vi "Add card dialog.vi"(8 "error in (no error)":errorcluster, 9 "Card Position":T1={"Rack #"=0, "Slot #"=1} {"Slot #" max=15}, 10 "Card Type in":string, 11 "Node Ptr":u64 format="%.0x") -> (0 "error out":errorcluster, 1 "Card Position out":T1={"Rack #"=0, "Slot #"=1} {"Slot #" max=15}, 2 "Name out":string, 3 "Node Ptr out":u64 format="%.0x", 4 "Cancelled?":bool)   [LabVIEW 2014, in "SLSC configuration System Explorer.lvlib"]
uses:
  SLSC configuration System Explorer.lvlib
  Type Defs/Card Position.ctl
  Shared/SPI Utility/Slot #.ctl
  Type Defs/Valid.ctl
  Shared/Constants.vi
  <vilib>/NI Veristand/Custom Device API/Custom Device API.lvlib
  Shared/SLSC configuration Shared.lvlib
panel:
  out "Valid?":T3
  in  "Name":string
  in  "Cancel":bool
  in  "Add":bool
  out "Card Type":string
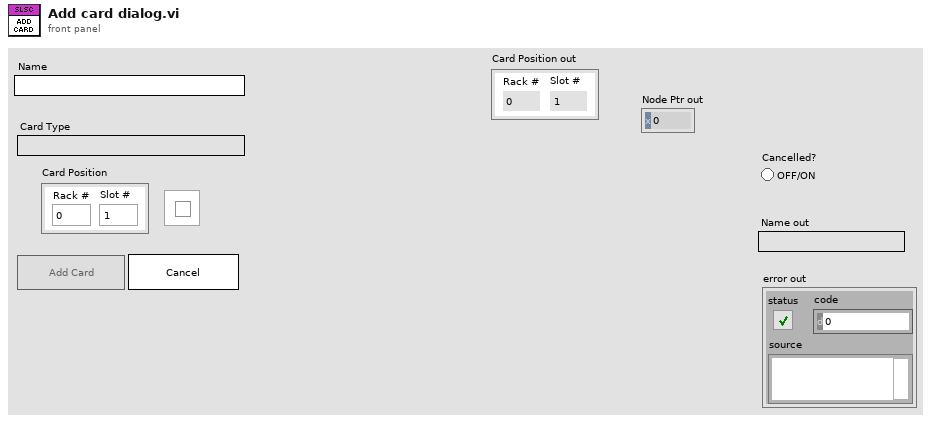
[diagram p1: front panel]
types:
  T1 = typedef "SLSC configuration Shared.lvlib/Card Position.ctl" = cluster{"Rack #":u8, "Slot #":T2}
  T2 = typedef "SLSC configuration Shared.lvlib/Slot #.ctl" = u8
  T3 = typedef "SLSC configuration System Explorer.lvlib/Valid.ctl" = bool
  T4 = enum8{"Enabled", "Disabled", "Disabled and Grayed Out"}
  T5 = typedef "Custom Device API.lvlib/Custom Device Item Ref.ctl" = u64
  T6 = typedef "Slot #.ctl" = u8
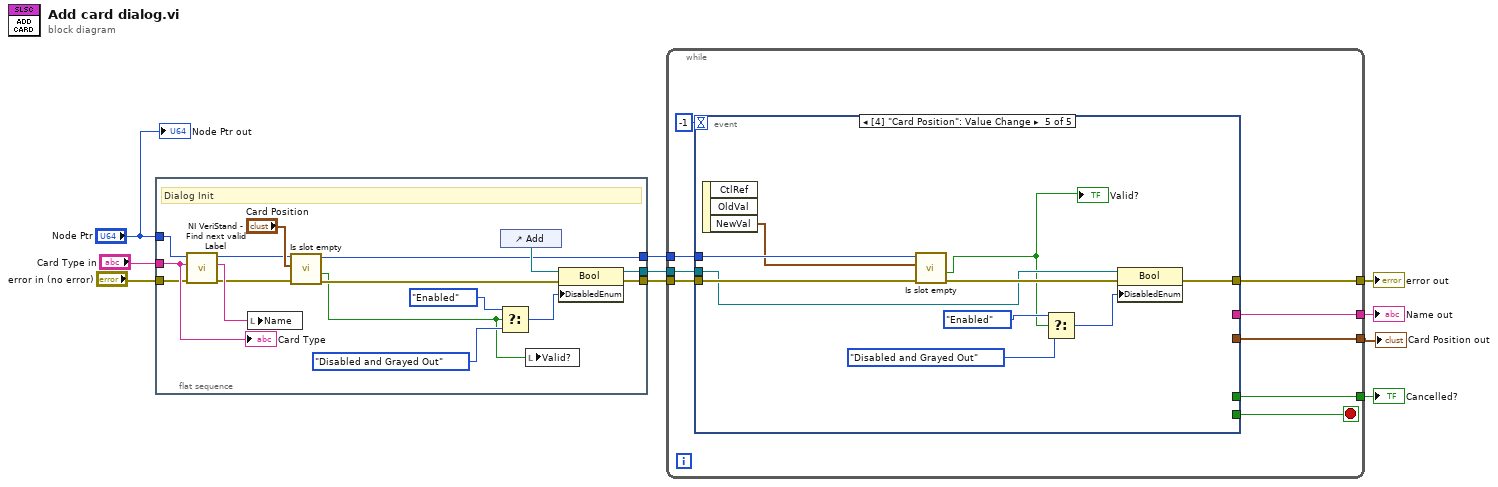
[diagram p0: block diagram]
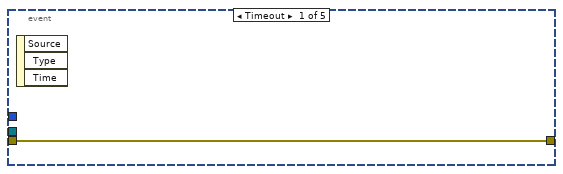
[diagram p2: hidden frame]
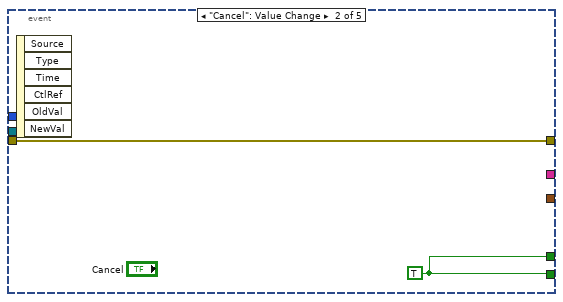
[diagram p3: hidden frame]
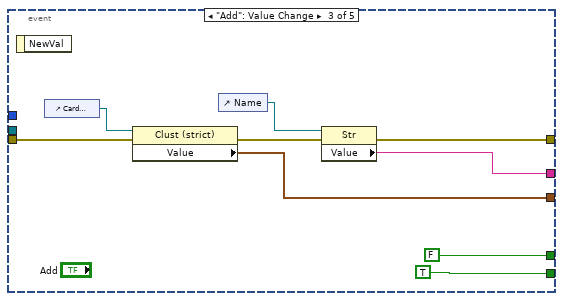
[diagram p4: hidden frame]
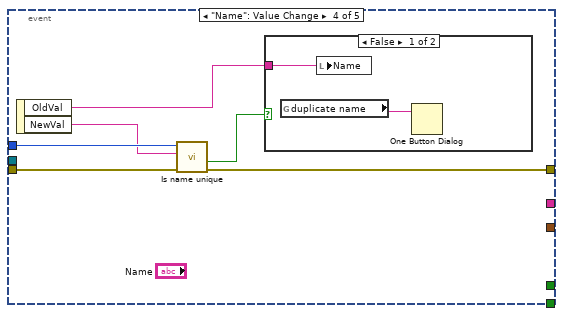
[diagram p5: hidden frame]
diagram:
  n1 = flat-sequence {
    tunnel: "Card Type in" -> [w26]
    tunnel: "error in (no error)" -> [w25]
    tunnel: "Node Ptr" -> [w21]
    tunnel: [w15] -> w7
    tunnel: [w23] -> w5
    tunnel: [w22] -> w4
    frame #0 {
      # "Dialog Init"
      n2 = call <vilib>:"NI VeriStand - Find next valid Label.vi"("error in (no error)"=w25, "Label"=w26, "Item Ref in"=w21) -> ("error out"=w19:errorcluster, "Label out"=w24:string, "Item Ref out"=w16:T5)  [unwired: 4 in, 2 out]
      n3 = local write "Name"(w24) -> ()
      n4 = call "Is slot empty.vi"("error in (no error)"=w19, "Card Position"="Card Position", "Devcie Ref in"=w16) -> ("error out"=w18:errorcluster, "Empty?"=w11:bool, "Device Ref out"=w15:T5)  [unwired: 6 in]
      n5 = Select(t=T4."Enabled" ("Disabled"), s=w11, f=T4."Disabled and Grayed Out" ("Disabled")) -> (s? t:f=w12:T4)
      n6 = control-ref of="Add"() -> (w20:refnum<vi>)
      n7 = local write "Valid?"(w11) -> ()
      n8 = property class="Bool"(reference=w20, error in=w18, "DisabledEnum"=w12) -> (reference out=w22:refnum<vi>, error out=w23:errorcluster)
      "Card Type" <- w26
    }
  }
  n9 = while {
    tunnel: w7 -> [w34]
    tunnel: w5 -> [w33]
    tunnel: [w32] -> w6
    tunnel: w4 -> [w31]
    tunnel: [w30] -> w3
    tunnel: [w28] -> w2
    tunnel: [w27] -> w1
    stop <- w35 stop-if-true
    n10 = event shown="[4] \"Card Position\": Value Change" {
      selector: _ -> [_ _ _ _ _]
      dyn-events: _ -> [_ _ _ _ _]
      timeout: -1 -> [_ _ _ _ _]
      tunnel: [_ w38 TRUE ("Cancel") _ _] -> w35
      tunnel: w34 -> [_ _ _ w52 w62]
      tunnel: w33 -> [w36 w37 w45 w51 w65]
      tunnel: [_ w38 FALSE ("Cancel") _ _] -> w32
      tunnel: w31 -> [_ _ _ _ w61]
      tunnel: [w36 w37 w42 w48 w63] -> w30
      tunnel: [_ _ w41 _ _] -> w28
      tunnel: [_ _ w40 _ _] -> w27
      event Timeout {
        n11 = event-data() -> ()  [unwired: 1 in, 3 out]
      }
      event "Cancel": Value Change {
        w38 = TRUE ("Cancel")
        n12 = event-data() -> ()  [unwired: 1 in, 6 out]
      }
      event "Add": Value Change {
        n13 = event-data() -> ()  [unwired: 1 in, 1 out]
        n14 = control-ref of="Card Position"() -> (w39:refnum<vi>)
        n15 = property class="Clust (strict)"(reference=w39, error in=w45) -> (error out=w44:errorcluster, "Value"=w40:cluster{"Rack #":u8, "Slot #":T6})  [unwired: 1 out]
        n16 = control-ref of="Name"() -> (w43:refnum<vi>)
        n17 = property class="Str"(reference=w43, error in=w44) -> (error out=w42:errorcluster, "Value"=w41:string)  [unwired: 1 out]
      }
      event "Name": Value Change {
        n18 = event-data() -> ("OldVal"=w53:string, "NewVal"=w49:string)  [unwired: 1 in]
        n19 = call "Is name unique.vi"("error in (no error)"=w51, "Name"=w49, "Device Ref in"=w52) -> ("error out"=w48:errorcluster, "Is name unique?"=w50:bool)  [unwired: 6 in, 1 out]
        n20 = case shown="False" w50 {
          tunnel: w53 -> [w55 _]
          frame False {
            n21 = global read "Constants.vi" "duplicate name"() -> (w54:string)
            n22 = local write "Name"(w55) -> ()
            n23 = One Button Dialog(message=w54) -> ()  [unwired: 1 in, 1 out]
          }
          frame True {
          }
        }
      }
      event Value Change {
        n24 = event-data() -> ("NewVal"=w60:T1)  [unwired: 1 in, 2 out]
        n25 = call "Is slot empty.vi"("error in (no error)"=w65, "Card Position"=w60, "Devcie Ref in"=w62) -> ("error out"=w64:errorcluster, "Empty?"=w56:bool)  [unwired: 6 in, 1 out]
        "Valid?" <- w56
        n26 = Select(t=T4."Enabled" ("Disabled"), s=w56, f=T4."Disabled and Grayed Out" ("Disabled")) -> (s? t:f=w57:T4)
        n27 = property class="Bool"(reference=w61, error in=w64, "DisabledEnum"=w57) -> (error out=w63:errorcluster)  [unwired: 1 out]
      }
    }
  }
  "Cancelled?" <- w6
  "error out" <- w3
  "Name out" <- w2
  "Card Position out" <- w1
  "Node Ptr out" <- "Node Ptr"
